vi "Shutdown User Event FGV.vi"(8 "error in":errorcluster, 11 "command":T1) -> (0 "error out":errorcluster, 3 "shutdown user event":refnum<user-event>)   [LabVIEW 2017]
doc: "This VI is a functional global variable used in every module for a correct shutdown procedure.\nFGV commands: Create, Get, Destroy"
uses:
  TypeDefs/Shutdown UE FGV Command.ctl
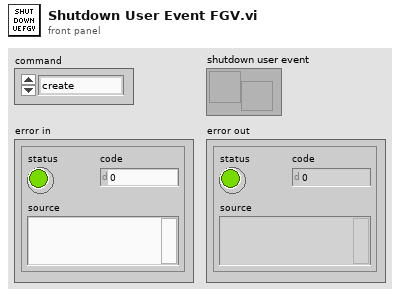
[diagram p1: front panel]
types:
  T1 = typedef "Shutdown UE FGV Command.ctl" = enum16{"create", "get", "destroy"}
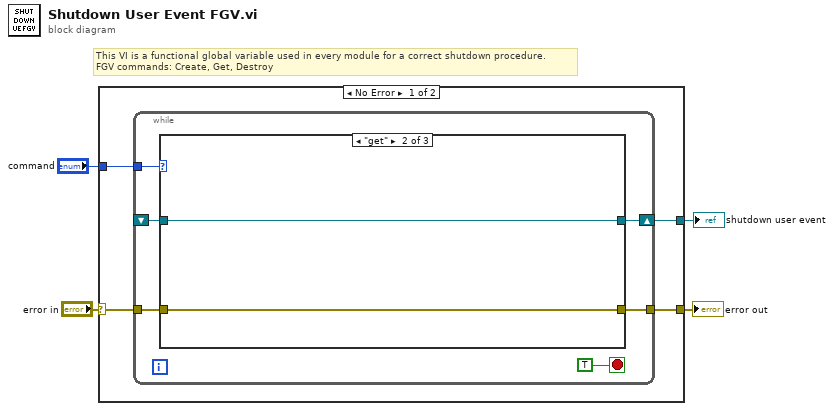
[diagram p0: block diagram]
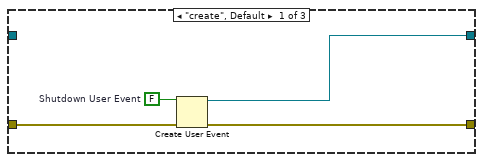
[diagram p2: hidden frame]
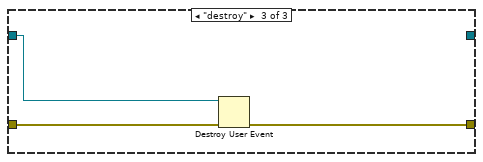
[diagram p3: hidden frame]
diagram:
  # "This VI is a functional global variable used in every module for a correct shutdown procedure.\nFGV commands: Create, Get, Destroy"
  n1 = case shown="No Error" "error in" {
    selector: "error in" -> [w8 w24]
    tunnel: [w7 w24] -> w3
    tunnel: "command" -> [w6 _]
    tunnel: [w5 _] -> w1
    frame No Error {
      n2 = while {
        tunnel: [w11] -> w7
        tunnel: w8 -> [w12]
        tunnel: w6 -> [w13]
        shift-right: [w10] -> w5
        shift-left: _ -> [w9]
        stop <- TRUE stop-if-true
        n3 = case shown="\"get\"" w13 {
          tunnel: w12 -> [w18 w20 w22]
          tunnel: [w17 w20 w21] -> w11
          tunnel: [w16 w19 _] -> w10
          tunnel: w9 -> [_ w19 w23]
          frame "create", Default {
            w15 = FALSE  # Shutdown User Event
            n4 = Create User Event(user event datatype=w15, error in=w18) -> (user event=w16:refnum<user-event>, error out=w17:errorcluster)
          }
          frame "get" {
          }
          frame "destroy" {
            n5 = Destroy User Event(user event=w23, error in=w22) -> (error out=w21:errorcluster)
          }
        }
      }
    }
    frame Error {
    }
  }
  "error out" <- w3
  "shutdown user event" <- w1
